vi "Launcher.vi"() -> ()   [LabVIEW 2020]
uses:
  LoadApp.vi
panel:
  in  "Run Demo?":bool
  out "Application Name":string
  out "Waiting Lights":T1
  out "Current Action":string caption="Current Action:"
  # "https://sites.psu.edu/hancocklab/"
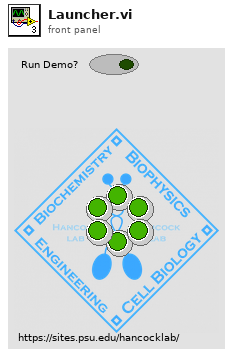
[diagram p1: front panel]
types:
  T1 = cluster{"wait 1":bool, "wait 2":bool, "wait 3":bool, "wait 4":bool, "wait 5":bool, "wait 6":bool}
  T2 = cluster{"[0]":bool, "[1]":bool, "[2]":bool, "[3]":bool, "[4]":bool, "[5]":bool}
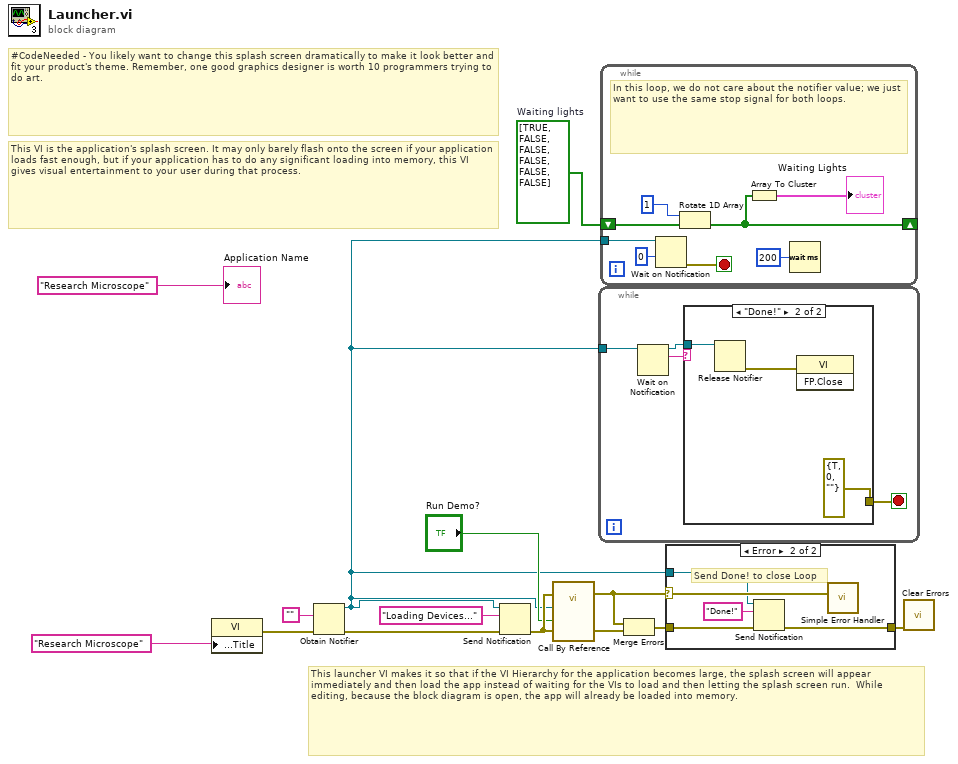
[diagram p0: block diagram]
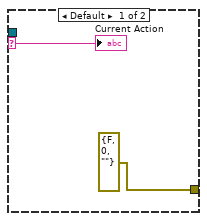
[diagram p3: hidden frame]
diagram:
  w10 = bool[] [TRUE, FALSE, FALSE, FALSE, FALSE, FALSE]  # Waiting lights
  # "#CodeNeeded - You likely want to change this splash screen dramatically to make it look better and fit your product's theme. Remember, one good graphics designer is worth 10 programmers trying to do art."
  # "This VI is the application's splash screen. It may only barely flash onto the screen if your application loads fast enough, but if your application has to do any significant loading into memory, this VI gives visual entertainment to your user during that process."
  # "This launcher VI makes it so that if the VI Hierarchy for the application becomes large, the splash screen will appear immediately and then load the app instead of waiting for the VIs to load and then letting the splash screen run.  While editing, because the block diagram is open, the app will already be loaded into memory."
  n1 = property class="VI"("Front Panel.Title"="Research Microscope" ("Window Title")) -> (error out=w14:errorcluster)  [unwired: 2 in, 1 out]
  n2 = Obtain Notifier(notification data type="", error in (no error)=w14) -> (notifier out=w1:refnum<notifier>, error out=w9:errorcluster)  [unwired: 2 in, 1 out]
  n3 = Send Notification(notification="Loading Devices...", notifier=w1, error in (no error)=w9) -> (error out=w5:errorcluster)  [unwired: 1 out]
  n4 = call-by-ref "?"(error in=w5, 3:"error in (no error)"=w5, "Demo?"="Run Demo?", "Status Notifier"=w1) -> (error out=w4:errorcluster, 0:"error out"=w6:errorcluster)  [unwired: 3 in, 1 out]
  n5 = while {
    tunnel: w1 -> [w18]
    stop <- w16 stop-if-true
    n6 = Wait on Notification(notifier=w18) -> (notifier out=w15:refnum<notifier>, notification=w17:string)  [unwired: 3 in, 2 out]
    n7 = case shown="\"Done!\"" w17 {
      selector: w17 -> [w20 _]
      tunnel: [errorcluster {"status"=FALSE, "code"=0, "source"=""} ("error IO") errorcluster {"status"=TRUE, "code"=0, "source"=""} ("error IO")] -> w16
      tunnel: w15 -> [_ w22]
      frame Default {
        "Current Action" <- w20
      }
      frame "Done!" {
        n8 = Release Notifier(notifier=w22) -> (error out=w21:errorcluster)  [unwired: 2 in, 2 out]
        n9 = invoke class="VI" method="FP.Close"(error in=w21) -> ()  [unwired: 2 in, 3 out]
      }
    }
  }
  n10 = while {
    shift-right: [w25] -> _
    shift-left: w10 -> [w27]
    tunnel: w1 -> [w29]
    stop <- w31 stop-if-true
    # "In this loop, we do not care about the notifier value; we just want to use the same stop signal for both loops."
    n11 = Wait on Notification(notifier=w29, timeout in ms (-1)=0) -> (error out=w31:errorcluster)  [unwired: 2 in, 3 out]
    n12 = Rotate 1D Array(1:w27, 2:1 ("n")) -> (0:w25:bool[])
    n13 = Array To Cluster(array=w25) -> (cluster=→"Waiting Lights":T2)
    n14 = Wait (ms)(milliseconds to wait=u32 200) -> ()  [unwired: 1 out]
  }
  n15 = Merge Errors(w4, w6) -> (w8:errorcluster)
  n16 = case shown="Error" w4 {
    tunnel: [w32 w35] -> w2
    tunnel: w8 -> [w32 w36]
    selector: w4 -> [_ w37]
    tunnel: w1 -> [_ w34]
    frame No Error {
    }
    frame Error {
      # "Send Done! to close Loop"
      n17 = Send Notification(notification="Done!", notifier=w34, error in (no error)=w36) -> (error out=w35:errorcluster)  [unwired: 1 out]
      n18 = call <vilib>:"Simple Error Handler.vi"("error in (no error)"=w37) -> ()  [unwired: 4 in, 5 out]
    }
  }
  n19 = call <vilib>:"Clear Errors.vi"("error in (no error)"=w2) -> ()  [unwired: 5 in, 2 out]
  "Application Name" <- "Research Microscope" ("Unlocalized")
